vi "F resp.vi"() -> ()   [LabVIEW 2020]
uses:
  <vilib>/measure/maspectr.llb/FFT Power Spectrum and PSD for 1 Chan.vi
  <vilib>/measure/NI_MAPro.lvlib
panel:
  out "Waveform Graph 2":cluster{"f0":dbl, "df":dbl, "magnitude":dbl[]}(graph)
  out "Frequency":dbl
  in  "sampling info":cluster{"Fs":dbl, "#s":dbl}={"Fs"=1000.0, "#s"=1000.0} {"Fs" format="%.2p"}
  in  "Steps":i32=128
  out "Waveform Graph":waveform(dbl)(graph)
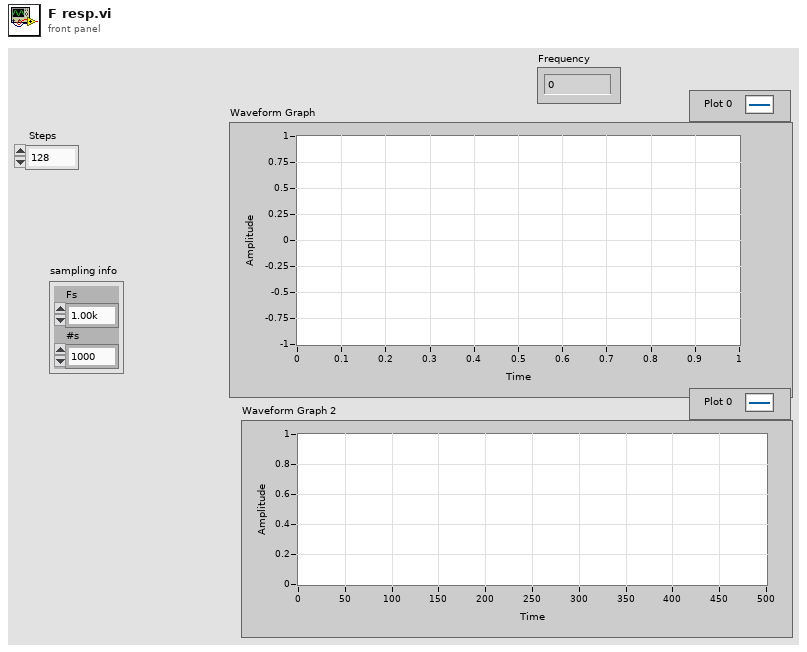
[diagram p1: front panel]
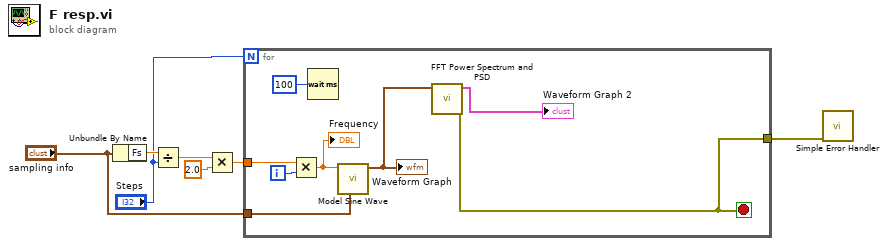
[diagram p0: block diagram]
diagram:
  n1 = Unbundle By Name("sampling info") -> ("Fs"=w6:dbl)
  n2 = Divide(x=w6, y="Steps") -> (x/y=w5:dbl)
  n3 = Multiply(x=w5, y=2.0) -> (x*y=w3:dbl)
  n4 = for {
    N: "Steps" -> [_]
    tunnel: "sampling info" -> [w11]
    tunnel: w3 -> [w15]
    tunnel: [w8] -> w1
    i -> [w14]
    stop <- w8 stop-if-true
    n5 = Multiply(x=w15, y=w14) -> (x*y=w12:dbl)
    "Frequency" <- w12
    n6 = Wait (ms)(milliseconds to wait=u32 100) -> ()  [unwired: 1 out]
    n7 = call "Model Sine Wave.vi"("sampling info"=w11, "Frequency"=w12) -> ("Waveform"=w10:waveform(dbl))  [unwired: 8 in, 1 out]
    "Waveform Graph" <- w10
    n8 = call-poly <vilib>:"FFT Power Spectrum and PSD.vi"("time signal"=w10) -> ("error out"=w8:errorcluster, "Power Spectrum / PSD"=→"Waveform Graph 2":cluster{"f0":dbl, "df":dbl, "magnitude":dbl[]})  [unwired: 7 in, 2 out]
  }
  n9 = call <vilib>:"Simple Error Handler.vi"("error in (no error)"=w1) -> ()  [unwired: 4 in, 5 out]
